vi "RenameFiles.vi"(3 "新油动机名称":string, 4 "旧油动机名称":string, 5 "Path":path) -> ()   [LabVIEW 2013]
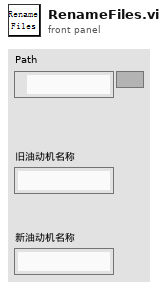
[diagram p1: front panel]
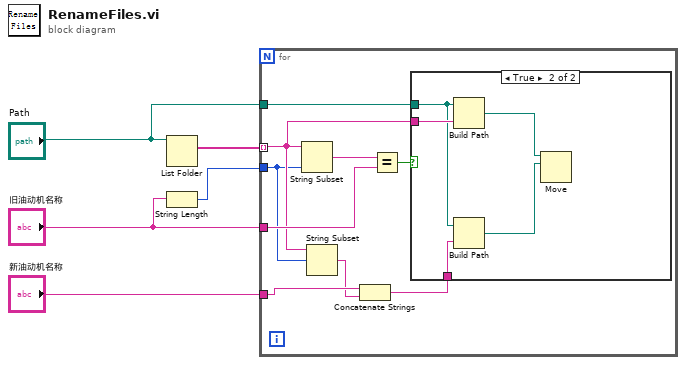
[diagram p0: block diagram]
diagram:
  n1 = List Folder(path="Path") -> (filenames=w5:string[])  [unwired: 3 in, 3 out]
  n2 = String Length(string="旧油动机名称") -> (length=w4:i32)
  n3 = for {
    tunnel: w5 -> [w10] mode=indexing
    tunnel: w4 -> [w9]
    tunnel: "旧油动机名称" -> [w13]
    tunnel: "Path" -> [w12]
    tunnel: "新油动机名称" -> [w8]
    n4 = String Subset(string=w10, length (rest)=w9) -> (substring=w14:string)  [unwired: 1 in]
    n5 = String Subset(string=w10, offset (0)=w9) -> (substring=w7:string)  [unwired: 1 in]
    n6 = Concatenate Strings(w8, w7) -> (w6:string)
    n7 = Equal?(x=w14, y=w13) -> (x = y?=w11:bool)
    n8 = case shown="True" w11 {
      tunnel: w12 -> [_ w17]
      tunnel: w10 -> [_ w19]
      tunnel: w6 -> [_ w16]
      frame False {
      }
      frame True {
        n9 = Build Path(base path=w17, name or relative path=w19) -> (appended path=w18:path)
        n10 = Build Path(base path=w17, name or relative path=w16) -> (appended path=w15:path)
        n11 = Move(source path=w18, 10:w15) -> ()  [unwired: 3 in, 3 out]
      }
    }
  }
